vi "Day10-04_QR 읽고 인터넷 연결.vi"() -> ()   [LabVIEW 2021]
uses:
  <vilib>/Platform/browser.llb/Open URL in Default Browser (string).vi
  <vilib>/vision/NI_Vision_Development_Module.lvlib
panel:
  out "Image":T1(plugin-control)
  out "Data":string
  in  "File Path":path
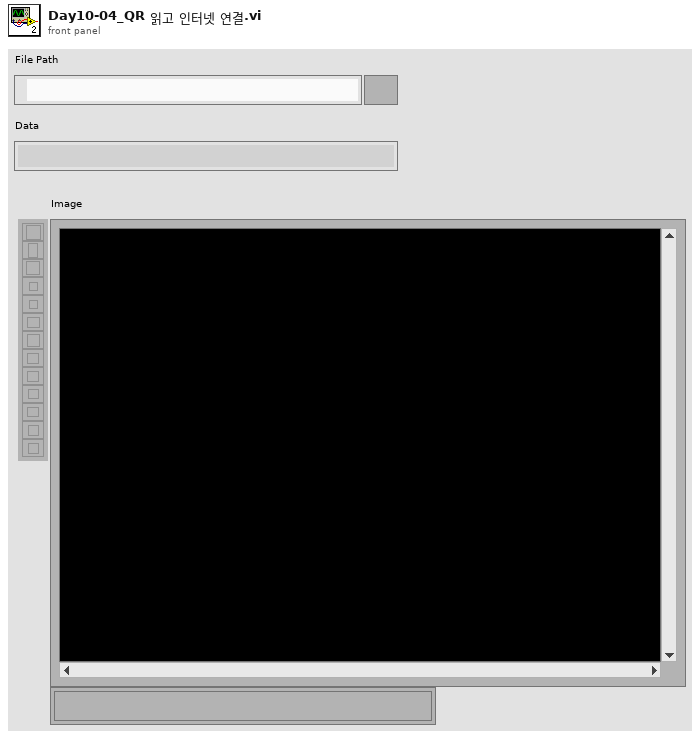
[diagram p1: front panel]
types:
  T1 = typedef "IMAQ Image.ctl" = refnum<image>
  T2 = typedef "QR Code Report.ctl" = cluster{"Found?":bool, "Data":string, "Bounding Box":cluster{"x":sgl, "y":sgl}[], "Errors Corrected":u32, "Dimensions (Rows/Cols)":u32, "Version":u32, "QR Model":T3, "Stream Mode":T4, "Barcode Polarity":T5, "Mirrored?":bool, "Append Stream Position":u32, "Size of Append Stream":u32, "First EAN-128 ID":i32, "First Alternate Language ID":i32, "Append Stream ID":u32, "Minimum Edge Strength":u32, "Demodulation Mode":T6, "Cell Sample Size":T7, "Cell Filter Mode":T8}
  T3 = typedef "QR Code Model Type.ctl" = i32
  T4 = typedef "QR Code Stream Mode Type.ctl" = i32
  T5 = typedef "Data Matrix Polarity.ctl" = i32
  T6 = typedef "Demodulation Mode.ctl" = i32
  T7 = typedef "Cell Sample Size.ctl" = i32
  T8 = typedef "Cell Filter Mode.ctl" = i32
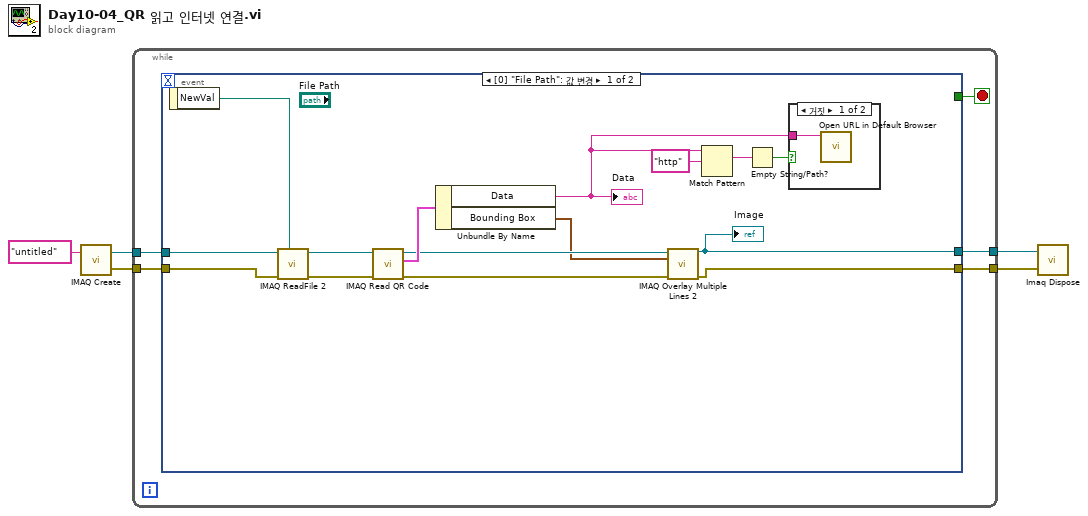
[diagram p0: block diagram]
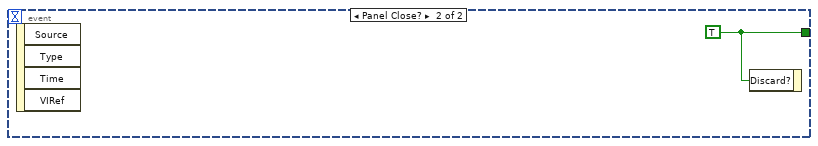
[diagram p3: hidden frame]
diagram:
  n1 = call "IMAQ Create"("Image Name"="untitled") -> ("New Image"=w5:T1, "error out"=w4:errorcluster)  [unwired: 3 in, 1 out]
  n2 = while {
    tunnel: w5 -> [w10]
    tunnel: w4 -> [w9]
    tunnel: [w7] -> w2
    tunnel: [w6] -> w1
    stop <- w8 stop-if-true
    n3 = event shown="[0] \"File Path\": 값 변경" {
      selector: _ -> [_ _]
      dyn-events: _ -> [_ _]
      timeout: _ -> [_ _]
      tunnel: w10 -> [w25 _]
      tunnel: w9 -> [w24 _]
      tunnel: [_ w27] -> w8
      tunnel: [w12 _] -> w7
      tunnel: [w11 _] -> w6
      event "File Path": Value Change {
        n4 = event-data() -> ("NewVal"=w23:path)  [unwired: 1 in]
        n5 = call "IMAQ ReadFile 2"("File Path"=w23, "error in (no error)"=w24, "Image"=w25) -> ("error out"=w21:errorcluster, "Image Out"=w22:T1)  [unwired: 4 in, 3 out]
        n6 = call "IMAQ Read QR Code"("error in (no error)"=w21, "Image"=w22) -> ("error out"=w18:errorcluster, "QR Code Report"=w20:T2, "Image (duplicate)"=w19:T1)  [unwired: 6 in, 1 out]
        n7 = Unbundle By Name(w20) -> ("Data"=w14:string, "Bounding Box"=w13:cluster{"x":sgl, "y":sgl}[])
        "Data" <- w14
        n8 = call "IMAQ Overlay Multiple Lines 2"("Image"=w19, "Line End Points"=w13, "error in (no error)"=w18) -> ("Image Out"=w12:T1, "error out"=w11:errorcluster)  [unwired: 11 in]
        "Image" <- w12
        n9 = Match Pattern(string=w14, regular expression="http" ("정규식")) -> (match substring=w17:string)  [unwired: 1 in, 3 out]
        n10 = Empty String/Path?(string/path=w17) -> (empty?=w15:bool)
        n11 = case shown="거짓" w15 {
          tunnel: w14 -> [w26 _]
          frame False {
            n12 = call-poly <vilib>:"Open URL in Default Browser.vi"("URL"=w26) -> ()  [unwired: 5 in, 2 out]
          }
          frame True {
          }
        }
      }
      event Panel Close? {
        w27 = TRUE
        n13 = event-data() -> ()  [unwired: 1 in, 4 out]
        n14 = event-data("Discard?"=w27) -> ()  [unwired: 1 in, 1 out]
      }
    }
  }
  n15 = call "Imaq Dispose"("Image"=w2, "error in (no error)"=w1) -> ()  [unwired: 4 in, 1 out]
